vi "Run_2_of_6_Tests.vi"() -> ()   [LabVIEW 2019]
uses:
  <vilib>/Rock Robotics/WPI/ThirdParty/JAS_Junk/TrajLib/Trajectory_Library.lvlib
panel:
  out "Meca Drive \nPose Est":bool
  out "Meca Drive \nOdometry":bool
  out "Meca Drive \nKinematics":bool
  out "String":string
  out "Flywheel Simulation":bool
  out "Matrix":bool
  out "PID":bool
  out "Math Utils":bool
  out "Linear Filter":bool
  out "Linear System Loop":bool
  out "All Tests Finished":bool
  out "Holonomic Drive Ctrl":bool
  out "Linear Plant Inv FF":bool
  out "Numerical Jacobian":bool
  out "Merwe Scaled Sigma Pts":bool
  out "Numerical Integration":bool
  out "Median Filter":bool
  out "Linear System ID":bool
  out "Kalman filter":bool
  out "PID Input / Output":bool
  out "Linear Quadradtic Regulator":bool
  # "FORMAL TRAJECTORY / CONTROL LIBRARY TEST PROCEDURE"
  # "FUNCTION NOT\nIMPLEMENTED"
  # "Extended Kalman Filter"
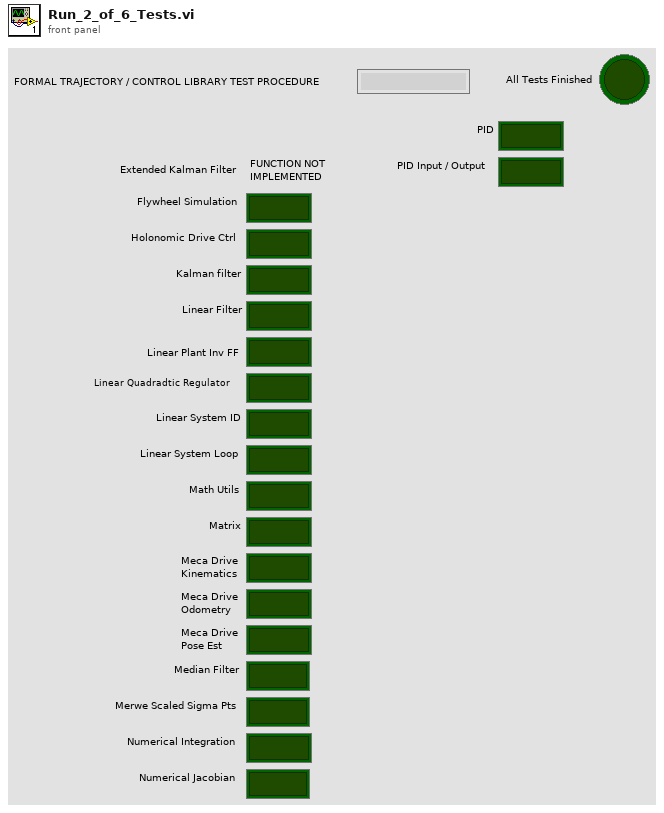
[diagram p1: front panel]
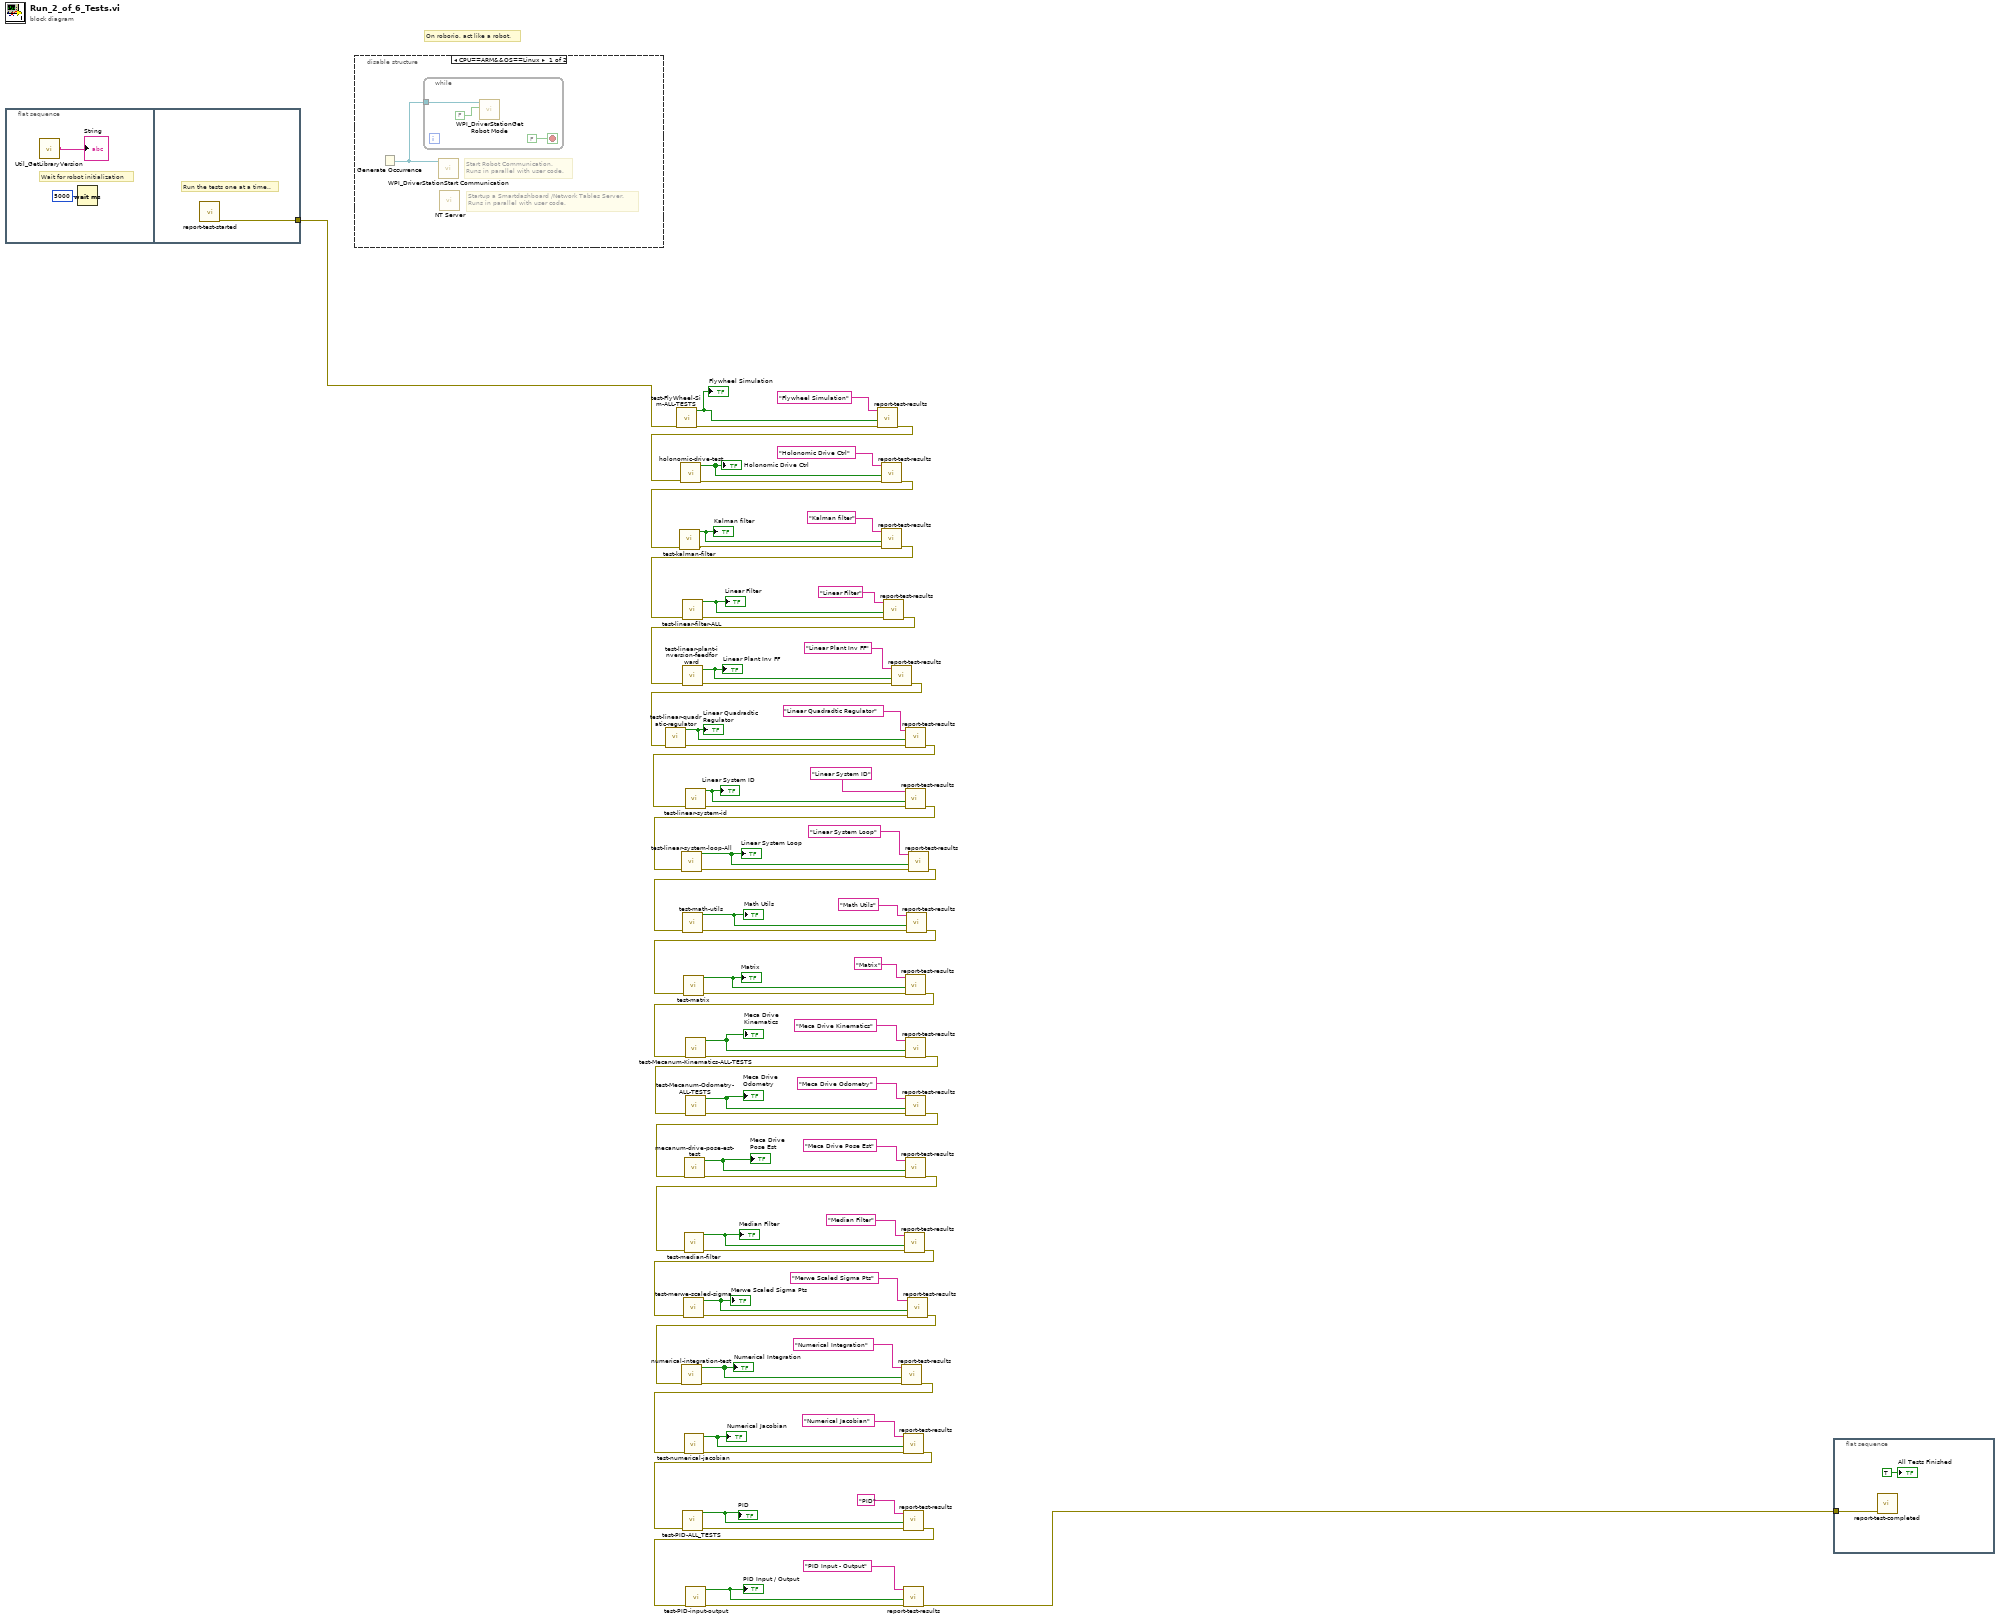
[diagram p0: block diagram]
diagram:
  # "On roborio, act like a robot."
  n1 = flat-sequence {
    tunnel: [w80] -> w1
    frame #0 {
      # "Wait for robot initialization"
      n2 = call <vilib>:"Util_GetLibraryVersion.vi"() -> ("TrajLibVersion"=→"String":string)  [unwired: 11 in]
      n3 = Wait (ms)(milliseconds to wait=u32 5000) -> ()  [unwired: 1 out]
    }
    frame #1 {
      # "Run the tests one at a time.."
      n4 = call "report-test-started.vi"() -> ("error out"=w80:errorcluster)  [unwired: 11 in]
    }
  }
  n5 = disable-structure shown="CPU==ARM&&OS==Linux" {
    frame condition #0 {
      # "Startup a Smartdashboard /Network Tables Server.\nRuns in parallel with user code."
      # "Start Robot Communication.\nRuns in parallel with user code."
      n6 = Generate Occurrence() -> (w81:refnum<k4>)
      n7 = while {
        tunnel: w81 -> [w84]
        stop <- FALSE stop-if-true
        n8 = call <vilib>:"WPI_DriverStationGet Robot Mode.vi"("Finish"=FALSE, "DS Occurrence"=w84) -> ()  [unwired: 10 out]
      }
      n9 = call <vilib>:"WPI_DriverStationStart Communication.vi"("occurrence"=w81) -> ()  [unwired: 2 in, 9 out]
      n10 = call <vilib>:"NT Server.vi"() -> ()  [unwired: 12 in]
    }
    frame condition #1 (active) {
    }
  }
  n11 = call "test-FlyWheel-Sim-ALL-TESTS.vi"("error in (no error)"=w1) -> ("error out"=w17:errorcluster, "All Passed"=w15:bool)  [unwired: 9 in]
  "Flywheel Simulation" <- w15
  n12 = call "report-test-results.vi"("error in (no error)"=w17, "TestPassed"=w15, "Test Name"="Flywheel Simulation") -> ("error out"=w16:errorcluster)  [unwired: 8 in]
  n13 = call "holonomic-drive-test.vi"("error in (no error)"=w16) -> ("error out"=w47:errorcluster, "ALL TESTS PASSED"=w75:bool)  [unwired: 9 in]
  "Holonomic Drive Ctrl" <- w75
  n14 = call "report-test-results.vi"("error in (no error)"=w47, "TestPassed"=w75, "Test Name"="Holonomic Drive Ctrl") -> ("error out"=w46:errorcluster)  [unwired: 8 in]
  n15 = call "test-kalman-filter.vi"("error in (no error)"=w46) -> ("error out"=w45:errorcluster, "ALL TESTS PASSED"=w74:bool)  [unwired: 9 in]
  "Kalman filter" <- w74
  n16 = call "report-test-results.vi"("error in (no error)"=w45, "TestPassed"=w74, "Test Name"="Kalman filter") -> ("error out"=w44:errorcluster)  [unwired: 8 in]
  n17 = call "test-linear-filter-ALL.vi"("error in (no error)"=w44) -> ("error out"=w42:errorcluster, "ALL TESTS GOOD"=w65:bool)  [unwired: 9 in]
  "Linear Filter" <- w65
  n18 = call "report-test-results.vi"("error in (no error)"=w42, "TestPassed"=w65, "Test Name"="Linear Filter") -> ("error out"=w41:errorcluster)  [unwired: 8 in]
  n19 = call "test-linear-plant-inversion-feedforward.vi"("error in (no error)"=w41) -> ("error out"=w40:errorcluster, "All Tests Passed"=w64:bool)  [unwired: 9 in]
  "Linear Plant Inv FF" <- w64
  n20 = call "report-test-results.vi"("error in (no error)"=w40, "TestPassed"=w64, "Test Name"="Linear Plant Inv FF") -> ("error out"=w39:errorcluster)  [unwired: 8 in]
  n21 = call "test-linear-quadratic-regulator.vi"("error in (no error)"=w39) -> ("error out"=w38:errorcluster, "ALL TESTS GOOD"=w63:bool)  [unwired: 9 in]
  "Linear Quadradtic Regulator" <- w63
  n22 = call "report-test-results.vi"("error in (no error)"=w38, "TestPassed"=w63, "Test Name"="Linear Quadradtic Regulator") -> ("error out"=w37:errorcluster)  [unwired: 8 in]
  n23 = call "test-linear-system-id.vi"("error in (no error)"=w37) -> ("error out"=w36:errorcluster, "All tests passed"=w62:bool)  [unwired: 9 in]
  "Linear System ID" <- w62
  n24 = call "report-test-results.vi"("error in (no error)"=w36, "TestPassed"=w62, "Test Name"="Linear System ID") -> ("error out"=w28:errorcluster)  [unwired: 8 in]
  n25 = call "test-linear-system-loop-All.vi"("error in (no error)"=w28) -> ("error out"=w29:errorcluster, "ALL TEsts Passed"=w61:bool)  [unwired: 9 in]
  "Linear System Loop" <- w61
  n26 = call "report-test-results.vi"("error in (no error)"=w29, "TestPassed"=w61, "Test Name"="Linear System Loop") -> ("error out"=w27:errorcluster)  [unwired: 8 in]
  n27 = call "test-math-utils.vi"("error in (no error)"=w27) -> ("error out"=w26:errorcluster, "ALL TESTS PASSED"=w60:bool)  [unwired: 9 in]
  "Math Utils" <- w60
  n28 = call "report-test-results.vi"("error in (no error)"=w26, "TestPassed"=w60, "Test Name"="Math Utils") -> ("error out"=w25:errorcluster)  [unwired: 8 in]
  n29 = call "test-matrix.vi"("error in (no error)"=w25) -> ("error out"=w30:errorcluster, "All Tests\nPassed"=w59:bool)  [unwired: 9 in]
  "Matrix" <- w59
  n30 = call "report-test-results.vi"("error in (no error)"=w30, "TestPassed"=w59, "Test Name"="Matrix") -> ("error out"=w11:errorcluster)  [unwired: 8 in]
  n31 = call "test-Mecanum-Kinematics-ALL-TESTS.vi"("error in (no error)"=w11) -> ("error out"=w13:errorcluster, "All Passed"=w12:bool)  [unwired: 9 in]
  "Meca Drive \nKinematics" <- w12
  n32 = call "report-test-results.vi"("error in (no error)"=w13, "TestPassed"=w12, "Test Name"="Meca Drive Kinematics") -> ("error out"=w7:errorcluster)  [unwired: 8 in]
  n33 = call "test-Mecanum-Odometry-ALL-TESTS.vi"("error in (no error)"=w7) -> ("error out"=w9:errorcluster, "All Passed"=w8:bool)  [unwired: 9 in]
  "Meca Drive \nOdometry" <- w8
  n34 = call "report-test-results.vi"("error in (no error)"=w9, "TestPassed"=w8, "Test Name"="Meca Drive Odometry") -> ("error out"=w3:errorcluster)  [unwired: 8 in]
  n35 = call "mecanum-drive-pose-est-test.vi"("error in (no error)"=w3) -> ("error out"=w5:errorcluster, "Test Passed"=w4:bool)  [unwired: 9 in]
  "Meca Drive \nPose Est" <- w4
  n36 = call "report-test-results.vi"("error in (no error)"=w5, "TestPassed"=w4, "Test Name"="Meca Drive Pose Est") -> ("error out"=w2:errorcluster)  [unwired: 8 in]
  n37 = call "test-median-filter.vi"("error in (no error)"=w2) -> ("error out"=w31:errorcluster, "ALL TESTS PASSED"=w58:bool)  [unwired: 9 in]
  "Median Filter" <- w58
  n38 = call "report-test-results.vi"("error in (no error)"=w31, "TestPassed"=w58, "Test Name"="Median Filter") -> ("error out"=w24:errorcluster)  [unwired: 8 in]
  n39 = call "test-merwe-scaled-sigma.vi"("error in (no error)"=w24) -> ("error out"=w32:errorcluster, "All Tests Passed"=w48:bool)  [unwired: 9 in]
  "Merwe Scaled Sigma Pts" <- w48
  n40 = call "report-test-results.vi"("error in (no error)"=w32, "TestPassed"=w48, "Test Name"="Merwe Scaled Sigma Pts") -> ("error out"=w23:errorcluster)  [unwired: 8 in]
  n41 = call "numerical-integration-test.vi"("error in (no error)"=w23) -> ("error out"=w33:errorcluster, "All passed"=w49:bool)  [unwired: 9 in]
  "Numerical Integration" <- w49
  n42 = call "report-test-results.vi"("error in (no error)"=w33, "TestPassed"=w49, "Test Name"="Numerical Integration") -> ("error out"=w22:errorcluster)  [unwired: 8 in]
  n43 = call "test-numerical-jacobian.vi"("error in (no error)"=w22) -> ("error out"=w34:errorcluster, "ALL Tests Passed"=w50:bool)  [unwired: 9 in]
  "Numerical Jacobian" <- w50
  n44 = call "report-test-results.vi"("error in (no error)"=w34, "TestPassed"=w50, "Test Name"="Numerical Jacobian") -> ("error out"=w21:errorcluster)  [unwired: 8 in]
  n45 = call "test-PID-ALL_TESTS.vi"("error in (no error)"=w21) -> ("error out"=w35:errorcluster, "All Passed"=w51:bool)  [unwired: 9 in]
  "PID" <- w51
  n46 = call "report-test-results.vi"("error in (no error)"=w35, "TestPassed"=w51, "Test Name"="PID") -> ("error out"=w20:errorcluster)  [unwired: 8 in]
  n47 = call "test-PID-input-output.vi"("error in (no error)"=w20) -> ("error out"=w43:errorcluster, "All Passed"=w52:bool)  [unwired: 9 in]
  "PID Input / Output" <- w52
  n48 = call "report-test-results.vi"("error in (no error)"=w43, "TestPassed"=w52, "Test Name"="PID Input - Output") -> ("error out"=w19:errorcluster)  [unwired: 8 in]
  n49 = flat-sequence {
    tunnel: w19 -> [w85]
    frame #0 {
      n50 = call "report-test-completed.vi"("error in (no error)"=w85) -> ()  [unwired: 10 in, 1 out]
      "All Tests Finished" <- TRUE ("All Tests Finished")
    }
  }
